vi "vms_registerCallback_M1M3.vi"(8 "error in (no error)":errorcluster, 10 "skipOld":bool, 11 "handle":i32) -> (0 "error out":errorcluster, 3 "function return":i32)   [LabVIEW 2016, in "SALLV_vms.lvlib"]
doc: "int vms_shm_registerCallback_M1M3LV(int handle, bool skipOld);"
uses:
  SALLV_vms.lvlib
  SALLV_vms.so
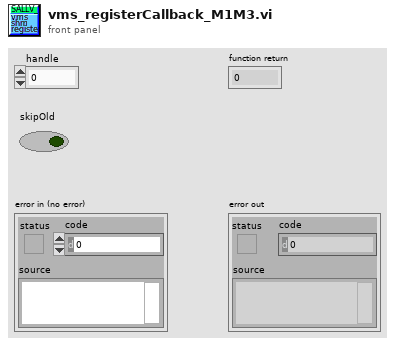
[diagram p1: front panel]
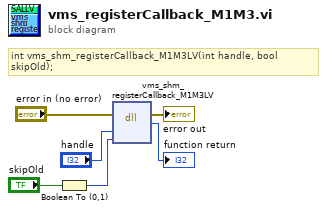
[diagram p0: block diagram]
diagram:
  # "int vms_shm_registerCallback_M1M3LV(int handle, bool skipOld);"
  n1 = Boolean To (0,1)(Boolean="skipOld") -> (0, 1=w3:i16)
  n2 = dll-call lib="opt/CODE/SALLV_vms/SALLV_vms.*" fn="vms_shm_registerCallback_M1M3LV"(error in="error in (no error)", "handle"="handle", "skipOld"=w3) -> (error out=→"error out":errorcluster, →"function return":i32)  [unwired: 4 in, 1 out]
